vi "design PID.vi"() -> ()   [LabVIEW 2017]
uses:
  <vilib>/addons/Control Design/_PID Design/Datatypes/cd_PID Gains.ctl
  <vilib>/addons/Control Design/_Model Construction/Model Creation.llb/Model Creation SubVI/cd_Create Transfer Function Model.vi
  <vilib>/addons/Control Design/_PID Design/cd_Design PID for Discrete Systems (TF).vi
  <vilib>/addons/Control Design/_PID Design/NI_CD_PID Design.lvlib
  <vilib>/addons/Control Design/_Model Construction/NI_LinSys_Model Creation.lvlib
panel:
  in  "approx pulse duration":dbl format="%#_13g"
  in  "target slope":dbl format="%#_13g"
  out "Design PID Gains":T1
  in  "lifetime":dbl format="%#_13g"
  in  "period":dbl format="%#_13g"
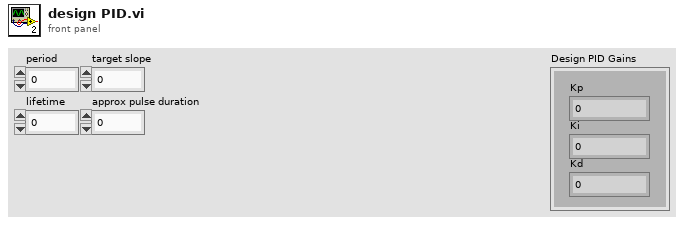
[diagram p1: front panel]
types:
  T1 = typedef "NI_CD_PID Design.lvlib/cd_PID Gains.ctl" = cluster{"Kp":dbl, "Ki":dbl, "Kd":dbl}
  T2 = typedef "NI_LinSys_Model Typedefs.lvlib/CD Transfer Function Model (MIMO).ctl" = cluster{"properties":T3, "transfer function(s)":T4[][]}
  T3 = typedef "NI_LinSys_Model Typedefs.lvlib/CD General Elements.ctl" = cluster{"Model name":string, "Input names":string[], "Output names":string[], "Input Delays":dbl[], "Output Delays":dbl[], "Sampling Time":dbl, "Notes":string}
  T4 = typedef "NI_LinSys_Model Typedefs.lvlib/CD Transfer Function Model (SISO).ctl" = cluster{"Numerator":dbl[], "Denominator":dbl[], "delay":dbl}
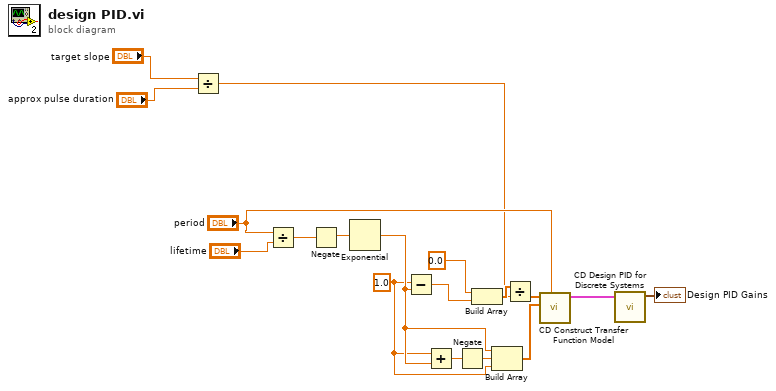
[diagram p0: block diagram]
diagram:
  w9 = 1.0
  n1 = Divide(x="target slope", y="approx pulse duration") -> (x/y=w1:dbl)
  n2 = Divide(x="period", y="lifetime") -> (x/y=w17:dbl)
  n3 = Negate(x=w17) -> (-x=w16:dbl)
  n4 = Exponential(1:w16) -> (0:w10:dbl)
  n5 = Subtract(x=w9, y=w10) -> (x-y=w14:dbl)
  n6 = Add(x=w9, y=w10) -> (x+y=w12:dbl)
  n7 = Negate(x=w12) -> (-x=w11:dbl)
  n8 = Build Array(0.0, w14) -> (w13:dbl[])
  n9 = Build Array(w10, w11, w9) -> (w8:dbl[])
  n10 = Divide(x=w13, y=w1) -> (x/y=w4:dbl[])
  n11 = call-poly <vilib>:"CD Construct Transfer Function Model.vi"("Sampling Time (s)"="period", "Denominator"=w8, "Numerator"=w4) -> ("Transfer Function Model"=w6:T2)  [unwired: 7 in, 1 out]
  n12 = call-poly <vilib>:"CD Design PID for Discrete Systems.vi"("Transfer Function Model"=w6) -> ("Design PID Gains"=→"Design PID Gains":T1)  [unwired: 7 in, 3 out]
